vi "Change System Configuration.vi"(6 "Subsystem I/O Attributes":T3[](array[typedef]), 8 "error in (no error)":errorcluster, 10 "Old System Configuration":T1, 11 "System Configuration":T1) -> (0 "error out":errorcluster, 2 "Succeed?":bool, 3 "dup System Configuration":T1)   [LabVIEW 2024]
doc: "Changes server configurations."
uses:
  Controls/Server/System Configuration.ctl
  Controls/Server/Subsystem Configuration.ctl
  Controls/Server/Subsystem IO Attributes.ctl
  Controls/Server/Subsystem IO Logging Attributes.ctl
  Controls/Server/Subsystem IO Alarm Attributes.ctl
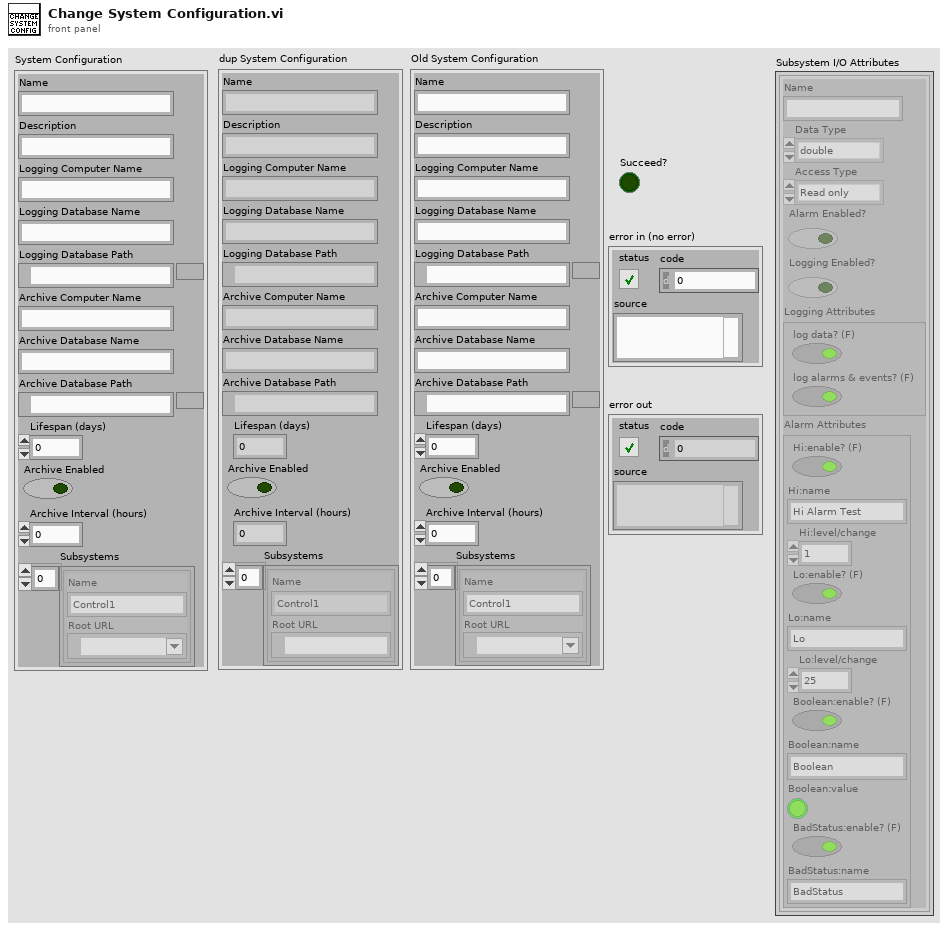
[diagram p1: front panel]
types:
  T1 = typedef "System Configuration.ctl" = cluster{"Name":string, "Description":string, "Logging Computer Name":string, "Logging Database Name":string, "Logging Database Path":path, "Archive Computer Name":string, "Archive Database Name":string, "Archive Database Path":path, "Lifespan (days)":u32, "Archive Enabled":bool, "Archive Interval (hours)":u32, "Subsystems":T2[]}
  T2 = typedef "Subsystem Configuration.ctl" = cluster{"Name":string, "Root URL":refnum<k21>}
  T3 = typedef "Subsystem IO Attributes.ctl" = cluster{"Name":string, "Data Type":enum32{"u32BitField", "bool", "double", "string", "int8", "uint8", "int16", "uint16", "int32", "uint32", "int64", "uint64", "single", "double waveform", "int16 waveform", "array of boolean", "array of int8", "array of uint8", "array of int16", "array of uint16", "array of int32", "array of uint32", "array of int64", "array of uint64", "array of single", "array of double", "array of double waveform", "array of int16 waveform", "array of string", "variant", "timestamp", "fixed point", "custom"}, "Access Type":enum32{"Read only", "Write only", "Read/write"}, "Alarm Enabled?":bool, "Logging Enabled?":bool, "Logging Attributes":T4, "Alarm Attributes":T5}
  T4 = typedef "Subsystem IO Logging Attributes.ctl" = cluster{"log data? (F)":bool, "log alarms & events? (F)":bool}
  T5 = typedef "Subsystem IO Alarm Attributes.ctl" = cluster{"Hi:enable? (F)":bool, "Hi:name":string, "Hi:level/change":dbl, "Lo:enable? (F)":bool, "Lo:name":string, "Lo:level/change":dbl, "Boolean:enable? (F)":bool, "Boolean:name":string, "Boolean:value":bool, "BadStatus:enable? (F)":bool, "BadStatus:name":string}
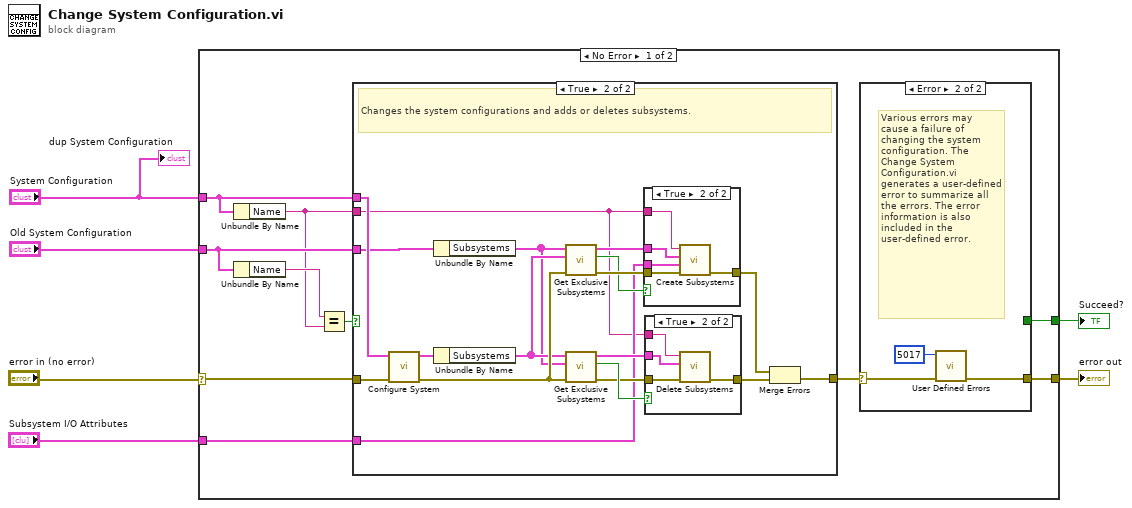
[diagram p0: block diagram]
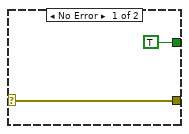
[diagram p2: hidden frame]
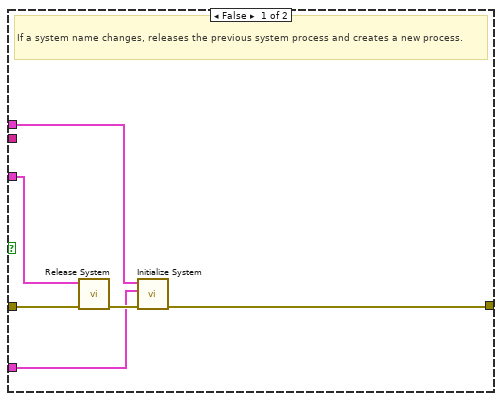
[diagram p3: hidden frame]
diagram:
  n1 = case shown="No Error" "error in (no error)" {
    selector: "error in (no error)" -> [w10 w57]
    tunnel: "Subsystem I/O Attributes" -> [w16 _]
    tunnel: [w8 w57] -> w5
    tunnel: "Old System Configuration" -> [w13 _]
    tunnel: "System Configuration" -> [w12 _]
    tunnel: [w7 _] -> w1
    frame No Error {
      n2 = Unbundle By Name(w12) -> ("Name"=w11:string)
      n3 = Unbundle By Name(w13) -> ("Name"=w14:string)
      n4 = Equal?(x=w14, y=w11) -> (x = y?=w15:bool)
      n5 = case shown="True" w15 {
        tunnel: w10 -> [w27 w45]
        tunnel: w12 -> [w23 w33]
        tunnel: [w24 w36] -> w9
        tunnel: w16 -> [w22 w34]
        tunnel: w13 -> [w26 w32]
        tunnel: w11 -> [_ w31]
        frame False {
          # "If a system name changes, releases the previous system process and creates a new process."
          n6 = call "Release System.vi"("error in (no error)"=w27, "System Configuration"=w26) -> ("error out"=w25:errorcluster)  [unwired: 9 in]
          n7 = call "Initialize System.vi"("error in (no error)"=w25, "Subsystem I/O Attributes"=w22, "System Configuration In"=w23) -> ("error out"=w24:errorcluster)  [unwired: 7 in, 1 out]
        }
        frame True {
          # "Changes the system configurations and adds or deletes subsystems."
          n8 = call "Configure System.vi"("error in (no error)"=w45, "System Configuration"=w33) -> ("error out"=w35:errorcluster, "dup System Configuration"=w30:T1)  [unwired: 8 in]
          n9 = Unbundle By Name(w32) -> ("Subsystems"=w28:T2[])
          n10 = Unbundle By Name(w30) -> ("Subsystems"=w29:T2[])
          n11 = call "Get Exclusive Subsystems.vi"("error in (no error)"=w35, "Subsystem Array B"=w29, "Subsystem Array A"=w28) -> ("error out"=w38:errorcluster, "Exist?"=w37:bool, "Exclusive Subsystems"=w39:T2[])  [unwired: 6 in]
          n12 = call "Get Exclusive Subsystems.vi"("error in (no error)"=w35, "Subsystem Array B"=w28, "Subsystem Array A"=w29) -> ("error out"=w40:errorcluster, "Exist?"=w43:bool, "Exclusive Subsystems"=w44:T2[])  [unwired: 6 in]
          n13 = case shown="True" w37 {
            tunnel: w38 -> [w51 w55]
            tunnel: w39 -> [_ w53]
            tunnel: [w51 w56] -> w42
            tunnel: w31 -> [_ w52]
            tunnel: w34 -> [_ w54]
            frame False {
            }
            frame True {
              n14 = call "Create Subsystems.vi"("error in (no error)"=w55, "Subsystem I/O Attributes"=w54, "Subsystems"=w53, "System Name"=w52) -> ("error out"=w56:errorcluster)  [unwired: 7 in]
            }
          }
          n15 = case shown="True" w43 {
            tunnel: w40 -> [w46 w49]
            tunnel: w44 -> [_ w48]
            tunnel: [w46 w50] -> w41
            tunnel: w31 -> [_ w47]
            frame False {
            }
            frame True {
              n16 = call "Delete Subsystems.vi"("error in (no error)"=w49, "Subsystems"=w48, "System Name"=w47) -> ("error out"=w50:errorcluster)  [unwired: 8 in]
            }
          }
          n17 = Merge Errors(w42, w41) -> (w36:errorcluster)
        }
      }
      n18 = case shown="Error" w9 {
        selector: w9 -> [w18 w20]
        tunnel: [w18 w19] -> w8
        tunnel: [TRUE ("Succeed?") _] -> w7
        frame No Error {
        }
        frame Error {
          # "Various errors may cause a failure of changing the system configuration. The Change System Configuration.vi generates a user-defined error to summarize all the errors. The error information is also included in the user-defined error."
          n19 = call "User Defined Errors.vi"("error in (no error)"=w20, "Error Code (0)"=5017 ("error code (0)")) -> ("error out"=w19:errorcluster)  [unwired: 9 in]
        }
      }
    }
    frame Error {
    }
  }
  "error out" <- w5
  "Succeed?" <- w1
  "dup System Configuration" <- "System Configuration"
